vi "p3.vi"() -> ()   [LabVIEW 2020]
panel:
  out "Data":dynamicdata(graph)
  out "Filtered PasaBajas":dynamicdata(graph) caption="Filtered Signal"
  out "Filtered PasaAltas":dynamicdata(graph) caption="Filtered Signal"
  in  "stop":bool
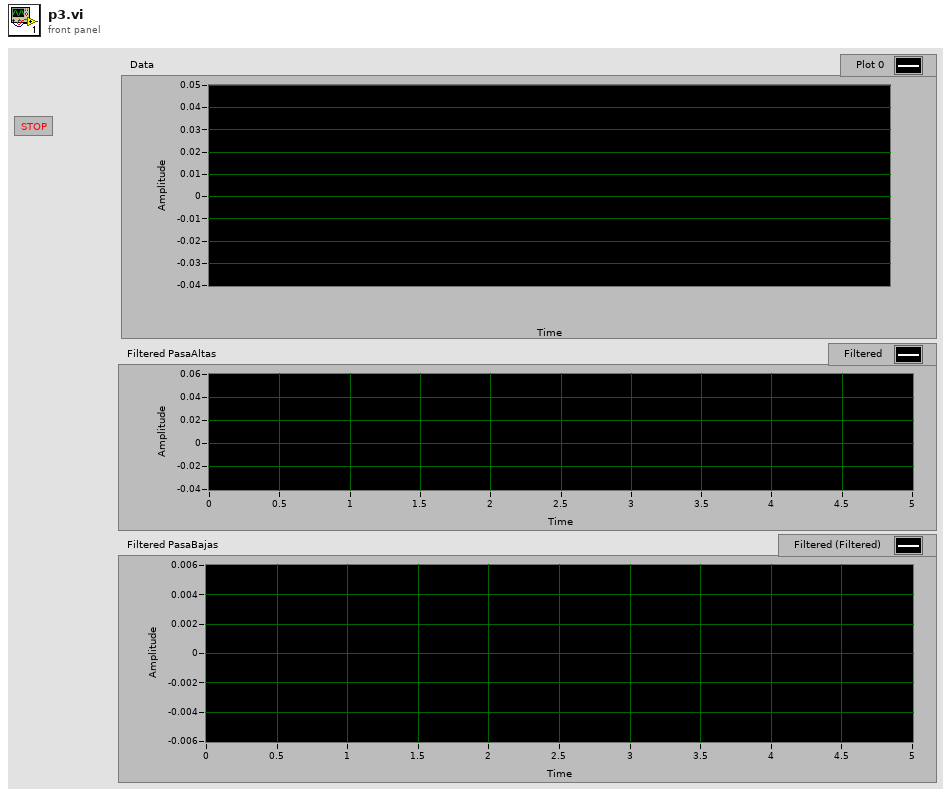
[diagram p1: front panel]
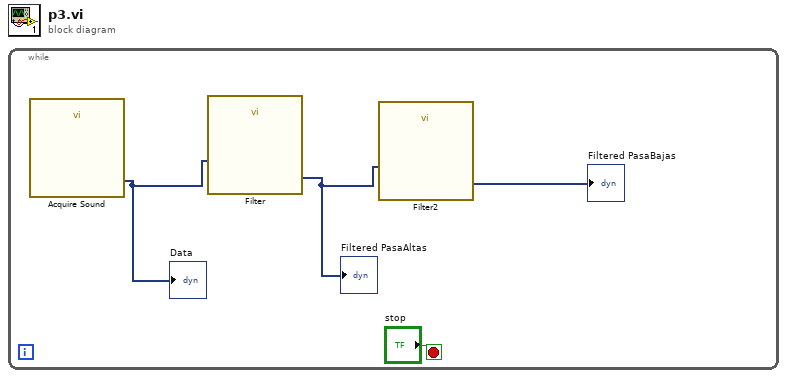
[diagram p0: block diagram]
diagram:
  n1 = while {
    stop <- "stop" stop-if-true
    n2 = call "Acquire Sound"() -> ("Data"=w1:dynamicdata)  [unwired: 18 in, 1 out]
    "Data" <- w1
    n3 = call "Filter"("Signal"=w1) -> ("Filtered Signal"=w2:dynamicdata)  [unwired: 9 in, 1 out]
    "Filtered PasaAltas" <- w2
    n4 = call "Filter2"("Signal"=w2) -> ("Filtered Signal"=→"Filtered PasaBajas":dynamicdata)  [unwired: 9 in, 1 out]
  }
